vi "LC Import.vi"(8 "error in (no error)":errorcluster caption="Error In") -> (0 "error out":errorcluster caption="Error Out")   [LabVIEW 2020]
uses:
  LC Mode.ctl
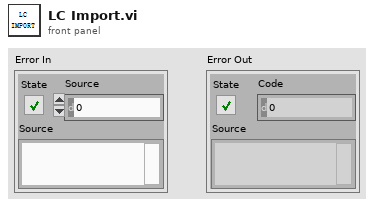
[diagram p1: front panel]
types:
  T1 = typedef "LC Mode.ctl" = enum16{"Init", "NONE", "Read", "Write", "Delete", "Clear", "Save"}
  T2 = cluster{"Read[0]":string, "Read[1]":string, "Read[2]":string, "Read[3]":string, "Read[4]":string, "Read[5]":string}
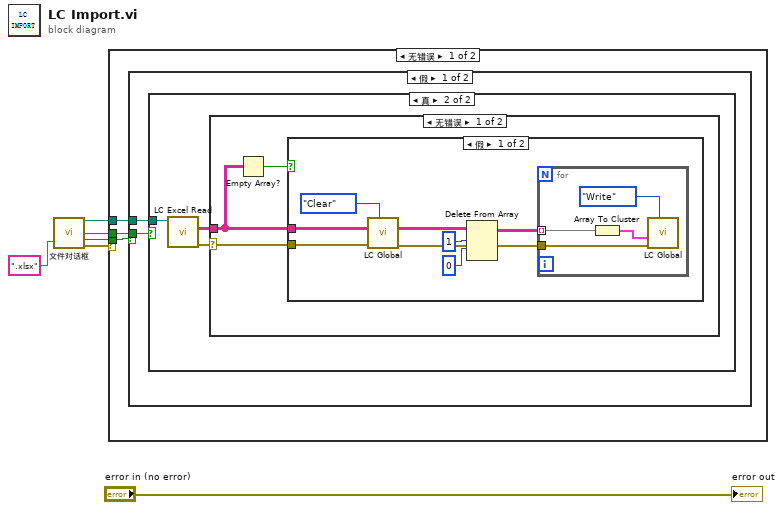
[diagram p0: block diagram]
diagram:
  n1 = call "文件对话框"("pattern (all files)"=".xlsx") -> ("selected path"=w2:path, "exists"=w1:bool, "cancelled"=w3:bool, "error out"=w5:errorcluster)  [unwired: 11 in]
  n2 = case shown="无错误" w5 {
    tunnel: w3 -> [w9 _]
    tunnel: w2 -> [w8 _]
    tunnel: w1 -> [w7 _]
    frame No Error {
      n3 = case shown="假" w9 {
        tunnel: w8 -> [w11 _]
        tunnel: w7 -> [w10 _]
        frame False {
          n4 = case shown="真" w10 {
            tunnel: w11 -> [_ w14]
            frame False {
            }
            frame True {
              n5 = call "LC Excel Read.vi"("Path"=w14) -> ("error out"=w12:errorcluster, "Read"=w13:string[][])  [unwired: 9 in]
              n6 = case shown="无错误" w12 {
                selector: w12 -> [w15 _]
                tunnel: w13 -> [w17 _]
                frame No Error {
                  n7 = Empty Array?(array=w17) -> (empty?=w16:bool)
                  n8 = case shown="假" w16 {
                    tunnel: w17 -> [w20 _]
                    tunnel: w15 -> [w19 _]
                    frame False {
                      n9 = call "LC Global.vi"("Mode"=LC_Mode."Clear", "error in (no error)"=w19) -> ("error out"=w18:errorcluster)  [unwired: 7 in, 2 out]
                      n10 = Delete From Array(array=w20, length=1 ("长度"), index (row)=0 ("索引 (行)")) -> (array with subset deleted=w22:string[][])  [unwired: 1 in, 1 out]
                      n11 = for {
                        tunnel: w22 -> [w27] mode=indexing
                        tunnel: w18 -> [w25]
                        n12 = Array To Cluster(array=w27) -> (cluster=w26:T2)
                        n13 = call "LC Global.vi"("Mode"=LC_Mode."Write", "error in (no error)"=w25, "Write"=w26) -> ()  [unwired: 6 in, 3 out]
                      }
                    }
                    frame True {
                    }
                  }
                }
                frame Error {
                }
              }
            }
          }
        }
        frame True {
        }
      }
    }
    frame Error {
    }
  }
  "error out" <- "error in (no error)"
